vi "Delete Tree Priv.vi"(8 "Error In":errorcluster, 10 "Unique ID":string, 11 "Tree Dictionary In":variant) -> (0 "Error Out":errorcluster, 3 "Tree Dictionary Out":variant)   [LabVIEW 2020, in "NI_VIAnCFGDataStructure.lvlib" / "Tree.lvclass"]
uses:
  <vilib>/addons/analyzer/VIAnCFGDataStructure/Tree Manager/Tree.lvclass
  <vilib>/addons/analyzer/VIAnCFGDataStructure/Tree Manager/Typedefs/Tree Cluster.ctl
  <vilib>/addons/analyzer/VIAnCFGDataStructure/Tree Data/Tree Data.lvclass
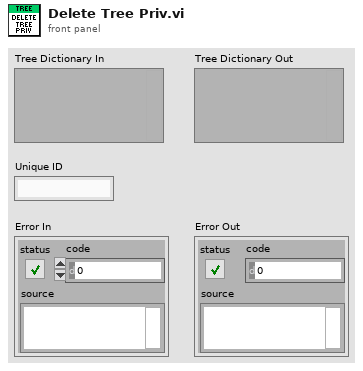
[diagram p1: front panel]
types:
  T1 = typedef "NI_VIAnCFGDataStructure.lvlib/Tree.lvclass/Tree Cluster.ctl" = cluster{"Unique ID":string, "Parent ID":string, "Child IDs":string[], "Name":string, "MetaData":string, "Data IDs":string[]}
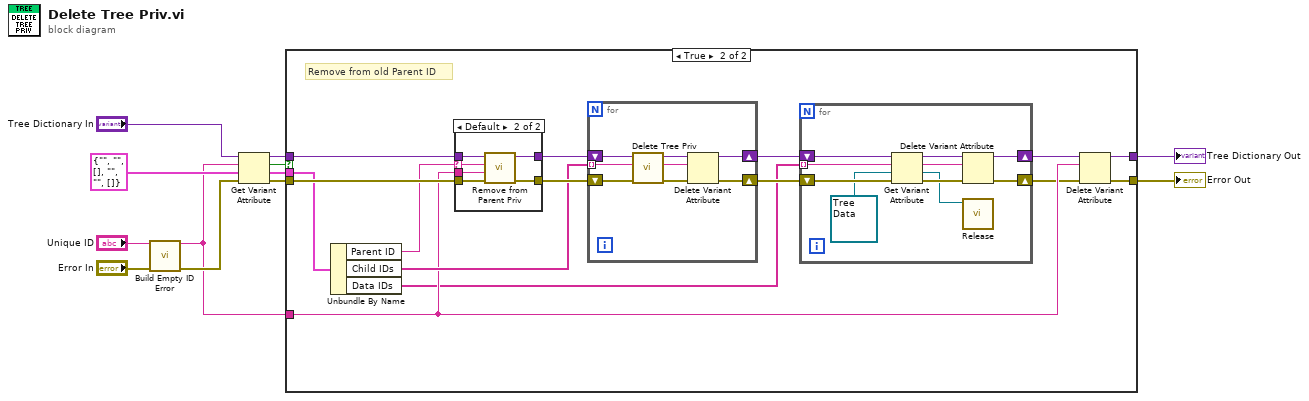
[diagram p0: block diagram]
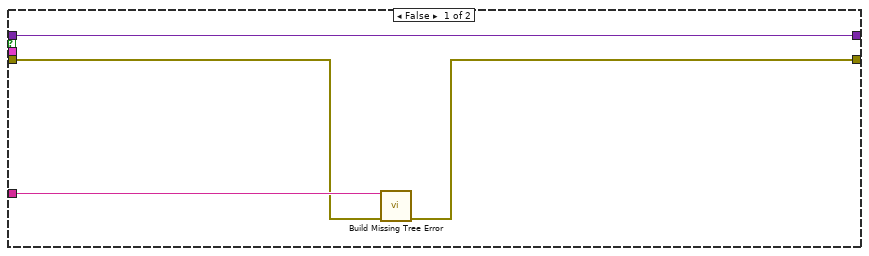
[diagram p2: hidden frame]
diagram:
  n1 = call <vilib>:"Build Empty ID Error.vi"("Unique ID"="Unique ID", "Error In"="Error In") -> ("Unique ID Out"=w1:string, "Error Out"=w2:errorcluster)  [unwired: 12 in]
  n2 = Get Variant Attribute(Variant="Tree Dictionary In", name=w1, default value (empty Variant)=T1 {"Unique ID"="", "Parent ID"="", "Child IDs"=[], "Name"="", "MetaData"="", "Data IDs"=[]} ("Cluster of class private data"), error in=w2) -> (duplicate Variant=w7:variant, found=w9:bool, value=w8:T1, error out=w6:errorcluster)
  n3 = case shown="True" w9 {
    tunnel: w8 -> [_ w30]
    tunnel: w7 -> [w16 w29]
    tunnel: w6 -> [w13 w31]
    tunnel: [w14 w25] -> w11
    tunnel: [w16 w24] -> w12
    tunnel: w1 -> [w15 w23]
    frame False {
      n4 = call <vilib>:"Build Missing Tree Error.vi"("Unique ID"=w15, "Error In"=w13) -> ("Error Out"=w14:errorcluster)  [unwired: 13 in]
    }
    frame True {
      # "Remove from old Parent ID"
      n5 = Unbundle By Name(w30) -> ("Parent ID"=w22:string, "Child IDs"=w26:string[], "Data IDs"=w17:string[])
      n6 = case shown="Default" w22 {
        selector: w22 -> [_ w43]
        tunnel: w31 -> [w41 w48]
        tunnel: w29 -> [w42 w47]
        tunnel: [w42 w46] -> w28
        tunnel: [w41 w45] -> w27
        tunnel: w23 -> [_ w44]
        frame "" {
        }
        frame Default {
          n7 = call <vilib>:"Remove from Parent Priv.vi"("Error In"=w48, "Unique ID"=w44, "Parent ID"=w43, "Tree Dictionary"=w47) -> ("Error Out"=w45:errorcluster, "Tree Dictionary Out"=w46:variant)  [unwired: 6 in]
        }
      }
      n8 = for {
        shift-right: [w50] -> w18
        shift-left: w27 -> [w54]
        shift-right: [w49] -> w21
        shift-left: w28 -> [w55]
        tunnel: w26 -> [w51] mode=indexing
        n9 = call <vilib>:"Delete Tree Priv.vi"("Error In"=w54, "Unique ID"=w51, "Tree Dictionary In"=w55) -> ("Error Out"=w52:errorcluster, "Tree Dictionary Out"=w53:variant)  [unwired: 7 in]
        n10 = Delete Variant Attribute(4:w52, 6:w51, 7:w53) -> (0:w50:errorcluster, 3:w49:variant)  [unwired: 1 out]
      }
      n11 = for {
        shift-right: [w33] -> w20
        shift-left: w21 -> [w40]
        shift-right: [w32] -> w19
        shift-left: w18 -> [w39]
        tunnel: w17 -> [w36] mode=indexing
        n12 = Get Variant Attribute(Variant=w40, name=w36, default value (empty Variant)=refnum<class "Tree Data.lvclass"> refnum ("Tree API.lvlib:Tree Data.lvclass"), error in=w39) -> (duplicate Variant=w38:variant, value=w34:refnum<class "Tree Data.lvclass">, error out=w35:errorcluster)  [unwired: 1 out]
        n13 = Delete Variant Attribute(4:w35, 6:w36, 7:w38) -> (0:w32:errorcluster, 3:w33:variant)  [unwired: 1 out]
        n14 = call-dynamic "Release.vi"("Tree Data"=w34) -> ()  [unwired: 10 in, 1 out]
      }
      n15 = Delete Variant Attribute(4:w19, 6:w23, 7:w20) -> (0:w25:errorcluster, 3:w24:variant)  [unwired: 1 out]
    }
  }
  "Tree Dictionary Out" <- w12
  "Error Out" <- w11
